vi "32xx_Init_COM.vi"(6 "Time\nOut (ms)":u32=7000 caption="timeout (ms)", 7 "Dupliquer\nla session (F)":bool, 8 "Entrée d'erreur":errorcluster={"status"=FALSE, "code"=0, "source"="L'opération s'est déroulée avec succès."}, 9 "Taille du\nbuffer \nd'entrée":u32=64 caption="Taille du buffer d'entrée", 10 "Mode d'accès":u32(ring) items=["Valeurs par défaut VISA"=0, "Verrouillage exclusif"=1, "Charger les paramètres configurés"=4], 11 "Port d'entrée":refnum<visa-resource-name>="COM5") -> (0 "Sortie d'erreur":errorcluster={"status"=FALSE, "code"=0, "source"="L'opération s'est déroulée avec succès."}, 3 "Port de sortie":refnum<visa-resource-name>="COM5", 5 "Config\nterminée ?":bool)   [LabVIEW 2020]
doc: "Initialisation de la session VISA (USB ou RS 232)"
panel:
  out "USB/RS Out":bool=TRUE
  in  "USB/RS (T:RS232)":bool caption="USB/RS232"
  in  "Param.\nsérie":T1={"Bauds"=9600, "bits"=8, "     Parité :"=enum."None", "bit(s) de stop"=10, "CTRL flux"=0} caption="Paramètres série" {"CTRL flux" items=["Aucun(e)"=0, "XON/XOFF"=1, "RTS/CTS"=2, "DTR/DSR"=4]; "bit(s) de stop" items=["1.0"=10, "2.0"=20]; "bits" min=5 max=8 step=1; "Bauds" items=["75"=75, "110"=110, "134"=134, "150"=150, "300"=300, "600"=600, "1200"=1200, "1800"=1800, "2400"=2400, "4800"=4800, "7200"=7200, "9600"=9600, "14400"=14400, "19200"=19200, "28800"=28800, "38400"=38400, "56000"=56000, "57600"=57600, "115200"=115200, "128000"=128000, "230400"=230400]}
  # "© 2020 elc CORPORATION.  \nALL RIGHTS RESERVED."
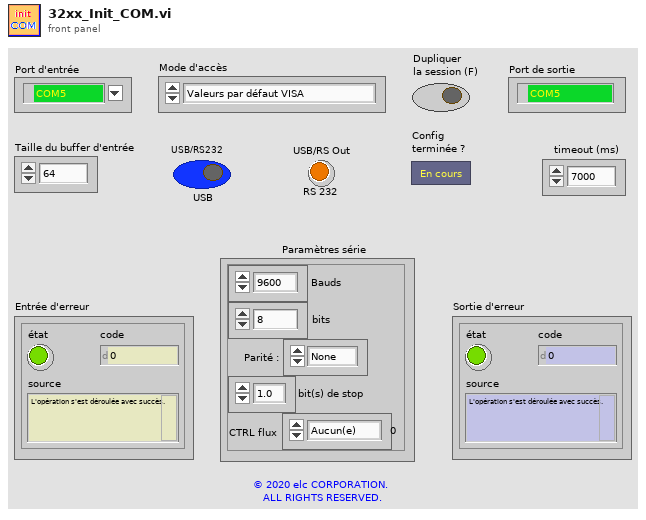
[diagram p1: front panel]
types:
  T1 = cluster{"Bauds":u32, "bits":u16, "     Parité :":enum16{"None", "Odd", "Even", "Mark", "Space"}, "bit(s) de stop":u16, "CTRL flux":u16}
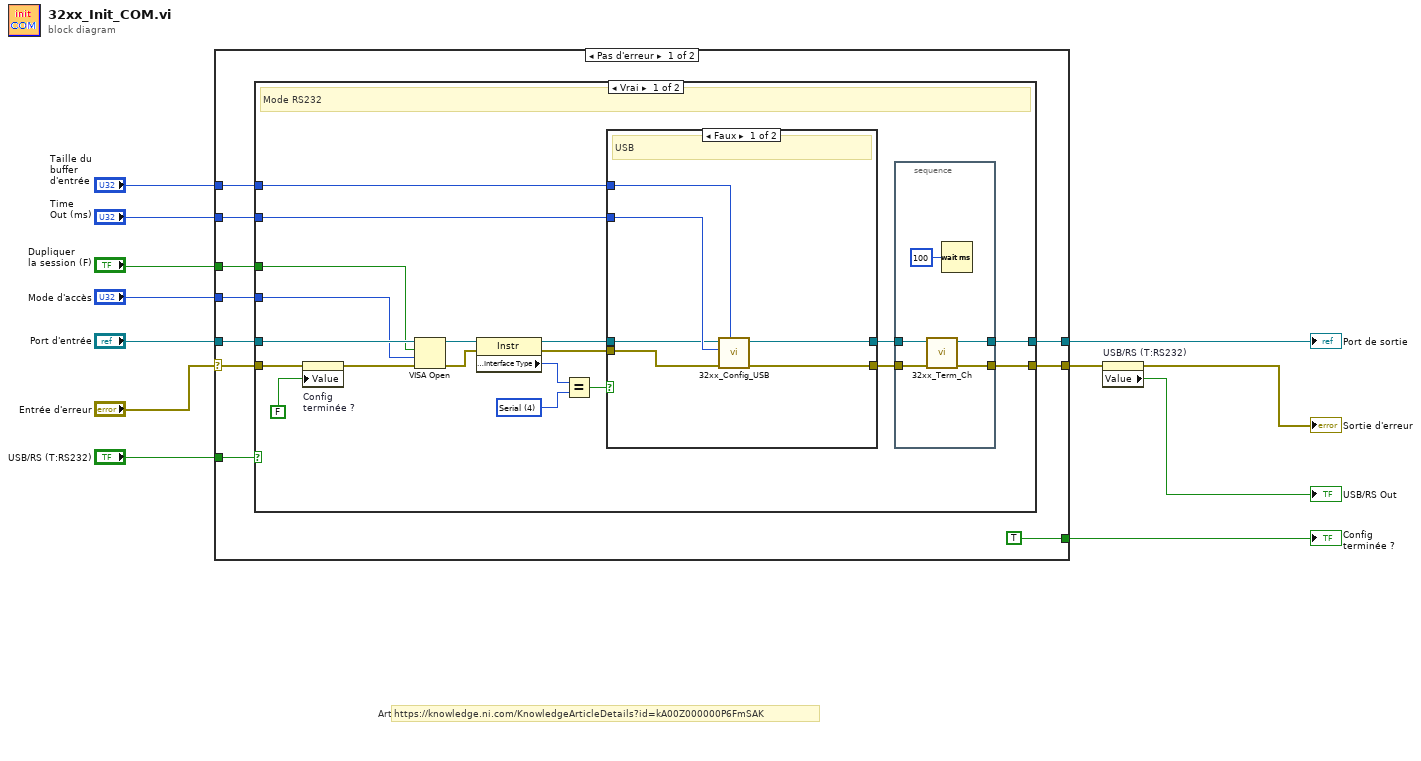
[diagram p0: block diagram]
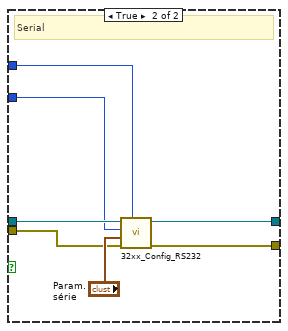
[diagram p2: hidden frame]
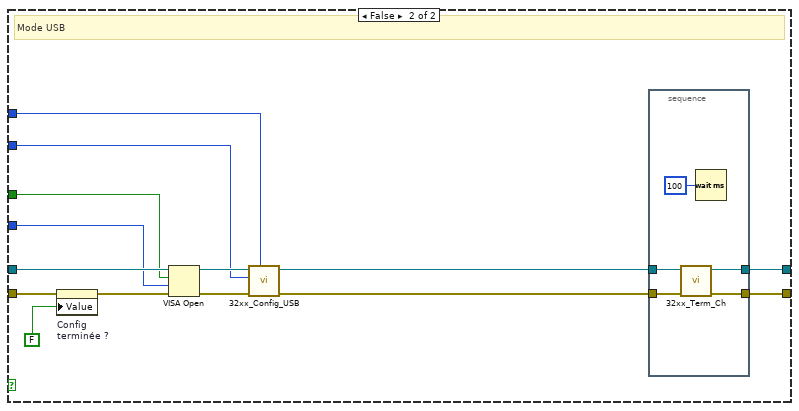
[diagram p3: hidden frame]
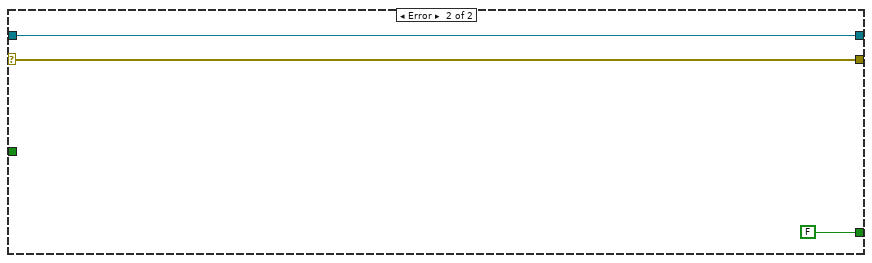
[diagram p4: hidden frame]
diagram:
  # "https://knowledge.ni.com/KnowledgeArticleDetails?id=kA00Z000000P6FmSAK"
  # "Article de labView au sujet  de l'erreur  -1073807298 & du Flush automatique :"
  n1 = case shown="Pas d'erreur" "Entrée d'erreur" {
    selector: "Entrée d'erreur" -> [w21 w80]
    tunnel: [w19 w80] -> w7
    tunnel: [w20 w81] -> w6
    tunnel: "Port d'entrée" -> [w22 w81]
    tunnel: "USB/RS (T:RS232)" -> [w18 _]
    tunnel: [TRUE ("Config\nterminée ?") FALSE ("Config\nterminée ?")] -> w5
    tunnel: "Mode d'accès" -> [w16 _]
    tunnel: "Taille du\nbuffer \nd'entrée" -> [w15 _]
    tunnel: "Dupliquer\nla session (F)" -> [w14 _]
    tunnel: "Time\nOut (ms)" -> [w13 _]
    frame No Error {
      n2 = case shown="Vrai" w18 {
        tunnel: w22 -> [w32 w71]
        tunnel: w21 -> [w31 w70]
        tunnel: [w30 w69] -> w20
        tunnel: [w29 w68] -> w19
        tunnel: w16 -> [w28 w67]
        tunnel: w15 -> [w25 w60]
        tunnel: w14 -> [w24 w66]
        tunnel: w13 -> [w23 w61]
        frame True {
          w39 = u16 4 items=["GPIB"=1, "VXI"=2, "GPIB-VXI"=3, "Serial"=4, "PXI"=5, "TCPIP"=6, "USB"=7] ("Interface Information:Interface Type")
          # "Mode RS232"
          n3 = property on="Config\nterminée ?" class="Bool (strict)"(error in=w31, "Value"=FALSE ("Config\nterminée ?")) -> (error out=w33:errorcluster)  [unwired: 1 in, 1 out]
          n4 = VISA Open(duplicate session (F)=w24, access mode=w28, error in (no error)=w33, VISA resource name=w32) -> (VISA resource name=w27:refnum<visa-resource-name>, error out=w26:errorcluster)  [unwired: 1 out]
          n5 = property class="Instr"(reference=w27, error in=w26) -> (reference out=w38:refnum<visa-resource-name>, error out=w37:errorcluster, "Interface Information:Interface Type"=w35:u16)
          n6 = Equal?(x=w35, y=w39) -> (x = y?=w36:bool)
          n7 = case shown="Faux" w36 {
            tunnel: [w46 w53] -> w41
            tunnel: [w47 w54] -> w40
            tunnel: w38 -> [w43 w51]
            tunnel: w37 -> [w42 w48]
            tunnel: w25 -> [w45 w52]
            tunnel: w23 -> [w44 w50]
            frame False {
              # "USB"
              n8 = call "32xx_Config_USB.vi"("Taille buffer d'entrée"=w45, "entrée d'erreur"=w42, "TimeOut (ms)"=w44, "Port Entrée"=w43) -> ("sortie d'erreur"=w46:errorcluster, "Port Sortie"=w47:refnum<visa-resource-name>)  [unwired: 6 in]
            }
            frame True {
              # "Serial"
              n9 = call "32xx_Config_RS232.vi"("Taille buffers E/S"=w52, "entrée d'erreur"=w48, "Paramètres série"="Param.\nsérie", "TimeOut (ms)"=w50, "Port Entrée"=w51) -> ("sortie d'erreur"=w53:errorcluster, "Port Sortie"=w54:refnum<visa-resource-name>)  [unwired: 5 in]
            }
          }
          n10 = stacked-sequence {
            tunnel: [w56] -> w30
            tunnel: w40 -> [w58]
            tunnel: [w55] -> w29
            tunnel: w41 -> [w57]
            frame #0 {
              n11 = call "32xx_Term_Ch.vi"("error in"=w57, "Visa In"=w58) -> ("error out"=w55:errorcluster, "Visa Out"=w56:refnum<visa-resource-name>)  [unwired: 8 in]
              n12 = Wait (ms)(milliseconds to wait=u32 100) -> ()  [unwired: 1 out]
            }
          }
        }
        frame False {
          # "Mode USB"
          n13 = property on="Config\nterminée ?" class="Bool (strict)"(error in=w70, "Value"=FALSE ("Config\nterminée ?")) -> (error out=w72:errorcluster)  [unwired: 1 in, 1 out]
          n14 = VISA Open(duplicate session (F)=w66, access mode=w67, error in (no error)=w72, VISA resource name=w71) -> (VISA resource name=w63:refnum<visa-resource-name>, error out=w62:errorcluster)  [unwired: 1 out]
          n15 = call "32xx_Config_USB.vi"("Taille buffer d'entrée"=w60, "entrée d'erreur"=w62, "TimeOut (ms)"=w61, "Port Entrée"=w63) -> ("sortie d'erreur"=w64:errorcluster, "Port Sortie"=w65:refnum<visa-resource-name>)  [unwired: 6 in]
          n16 = stacked-sequence {
            tunnel: [w77] -> w69
            tunnel: w65 -> [w75]
            tunnel: [w76] -> w68
            tunnel: w64 -> [w74]
            frame #0 {
              n17 = call "32xx_Term_Ch.vi"("error in"=w74, "Visa In"=w75) -> ("error out"=w76:errorcluster, "Visa Out"=w77:refnum<visa-resource-name>)  [unwired: 8 in]
              n18 = Wait (ms)(milliseconds to wait=u32 100) -> ()  [unwired: 1 out]
            }
          }
        }
      }
    }
    frame Error {
    }
  }
  "Port de sortie" <- w6
  "Config\nterminée ?" <- w5
  n19 = property on="USB/RS (T:RS232)" class="Bool (strict)"(error in=w7) -> (error out=→"Sortie d'erreur":errorcluster, "Value"=→"USB/RS Out":bool)  [unwired: 1 in, 1 out]
